vi "ValidateVariableJSON.vi"(8 "error in (no error)":errorcluster, 10 "JSON Variable Object":string) -> (0 "error out":errorcluster, 1 "JSON Error String":string, 2 "Valid?":bool)   [LabVIEW 2013]
uses:
  JSONVariable.ctl
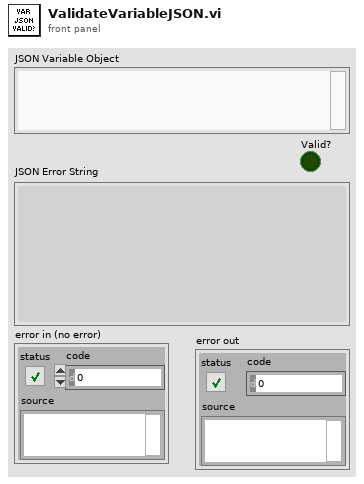
[diagram p1: front panel]
types:
  T1 = typedef "JSONVariable.ctl" = cluster{"name":string, "defaultValue":dbl, "sequenceFunction":string, "informIgor":bool, "sequence":bool}
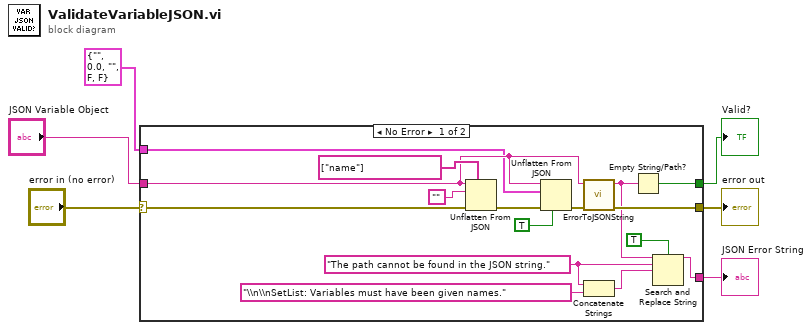
[diagram p0: block diagram]
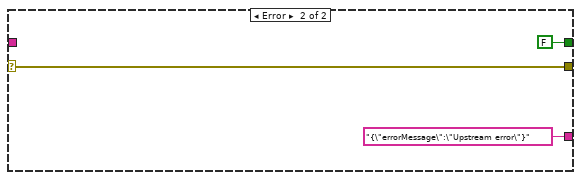
[diagram p2: hidden frame]
diagram:
  n1 = case shown="No Error" "error in (no error)" {
    selector: "error in (no error)" -> [w18 w25]
    tunnel: T1 {"name"="", "defaultValue"=0.0, "sequenceFunction"="", "informIgor"=FALSE, "sequence"=FALSE} ("JSONVariable") -> [w14 _]
    tunnel: "JSON Variable Object" -> [w15 _]
    tunnel: [w12 "{\"errorMessage\":\"Upstream error\"}" ("JSON string")] -> w4
    tunnel: [w20 FALSE] -> w3
    tunnel: [w19 w25] -> w1
    frame No Error {
      w9 = "The path cannot be found in the JSON string." ("search string")
      n2 = Unflatten From JSON(path=string[] ["name"], JSON string=w15, type and defaults="", error in (no error)=w18) -> (error out=w16:errorcluster)  [unwired: 3 in, 1 out]
      n3 = Unflatten From JSON(JSON string=w15, type and defaults=w14, default null elements? (F)=TRUE, error in (no error)=w16) -> (error out=w21:errorcluster)  [unwired: 3 in, 1 out]
      n4 = call "ErrorToJSONString.vi"("error in (no error)"=w21, "problemJSON"=w15) -> ("error out"=w19:errorcluster, "JSON Error string"=w13:string)  [unwired: 8 in]
      n5 = Concatenate Strings(w9, "\\n\\nSetList: Variables must have been given names." ("string")) -> (w10:string)
      n6 = Empty String/Path?(string/path=w13) -> (empty?=w20:bool)
      n7 = Search and Replace String(case sensitive?=TRUE ("ignore case? (F)"), input string=w13, search string=w9, replace string=w10) -> (result string=w12:string)  [unwired: 4 in, 3 out]
    }
    frame Error {
    }
  }
  "JSON Error String" <- w4
  "Valid?" <- w3
  "error out" <- w1
